vi "OP400ZP_prep bdd Type.vi"(8 "tabin":string[](array[string]), 11 "type":i32) -> (0 "Tableau":string[](array[string]))   [LabVIEW 2020]
uses:
  OP400ZP_selectdata.ctl
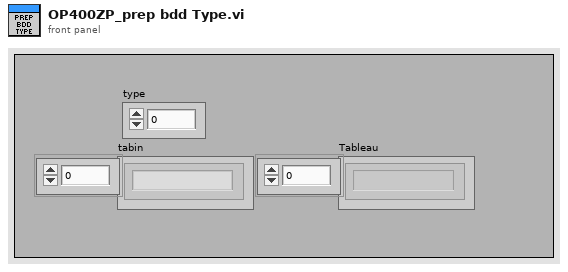
[diagram p1: front panel]
types:
  T1 = typedef "OP400ZP_selectdata.ctl" = u16
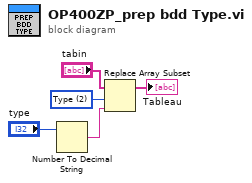
[diagram p0: block diagram]
diagram:
  w1 = T1 2 items=["IdOp400", "SN", "Type", "DateStart", "OCV", "ACIR", "InsuP", "InsuN", "TC0", "TC1", "DeltaTC", "VC0", "VC1", "DeltaVC", "MCU", "Tfactory", "RefLimite", "IniFileVers", "SoftVers", "ImageVers", "Pass", "Operateur", "TempsTest"] ("Menu déroulant")
  n1 = Number To Decimal String(number="type") -> (decimal integer string=w3:string)  [unwired: 1 in]
  n2 = Replace Array Subset(array="tabin", new element=w3, index=w1) -> (→"Tableau":string[])
